vi "Get Channels.vi"(11 "Perform Action on Const Channel Strategy in":refnum<class "Perform Action on N Const Channels Strategy.lvclass">) -> (2 "Channels":string[](array[string]), 3 "Perform Action on Const Channel Strategy out":refnum<class "Perform Action on N Const Channels Strategy.lvclass">)   [LabVIEW 2024, in "HAL.lvlib" / "Perform Action on N Const Channels Strategy.lvclass"]
uses:
  Perform Action on N Const Channels Strategy.lvclass
  Perform Action on N Const Channels Strategy.lvclass/Perform Action on N Const Channels Strategy.ctl
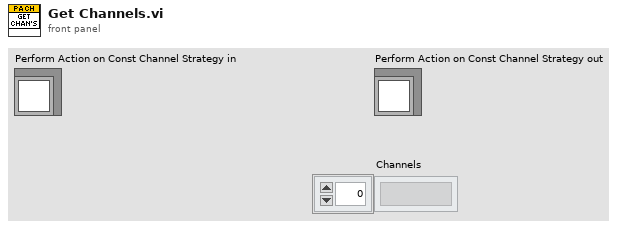
[diagram p1: front panel]
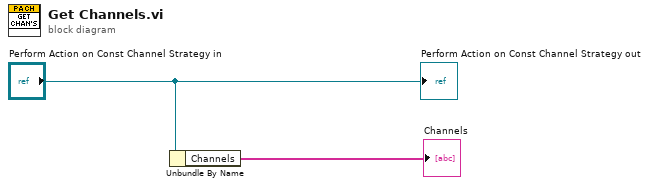
[diagram p0: block diagram]
diagram:
  n1 = Unbundle By Name("Perform Action on Const Channel Strategy in") -> ("Channels"=→"Channels":string[])
  "Perform Action on Const Channel Strategy out" <- "Perform Action on Const Channel Strategy in"
